vi "Stop Core.vi"(10 "final error code":i32, 11 "Nested in":refnum<class "[V] Waveform.lvclass">) -> (3 "Nested out":refnum<class "[V] Waveform.lvclass">)   [LabVIEW 2020, in "[V] Waveform.lvlib" / "[V] Waveform.lvclass"]
doc: "(<B>Filename</B>: Actor Framework.lvlib:Actor.lvclass:Stop Core.vi)\n\nDefines what the actor does before it stops. Use the <B>final error code</B> input to determine whether the actor shut down in response to an error.\n\nBy default, this method does nothing. A descendant class may override it to define behavior, such as shutting down any processes the actor initiated in its override of the Actor Core method."
uses:
  [V] Waveform.lvclass
  <vilib>/ActorFramework/Actor/Actor.lvclass
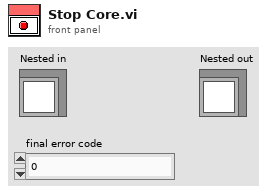
[diagram p1: front panel]
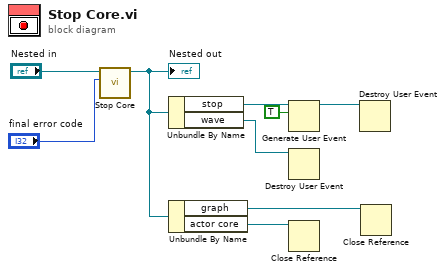
[diagram p0: block diagram]
diagram:
  n1 = call-parent "Stop Core.vi"("final error code"="final error code", "Actor in"="Nested in") -> ("Actor out"=w3:refnum<class "[V] Waveform.lvclass">)  [unwired: 9 in]
  "Nested out" <- w3
  n2 = Unbundle By Name ("Unbundle Events")(w3) -> ("stop"=w5:refnum<user-event>, "wave"=w4:refnum<user-event>)
  n3 = Unbundle By Name ("Unbundle Events")(w3) -> ("graph"=w1:refnum<vi>, "actor core"=w2:refnum<vi>)
  n4 = Generate User Event(user event=w5, event data cluster=TRUE ("event data")) -> (user event out=w6:refnum<user-event>)  [unwired: 2 in, 1 out]
  n5 = Destroy User Event(user event=w4) -> ()  [unwired: 1 in, 1 out]
  n6 = Close Reference(reference=w2) -> ()  [unwired: 1 in, 1 out]
  n7 = Destroy User Event(user event=w6) -> ()  [unwired: 1 in, 1 out]
  n8 = Close Reference(reference=w1) -> ()  [unwired: 1 in, 1 out]
